vi "statemachine.vi"() -> ()   [LabVIEW 2025]
uses:
  Control 1.ctl
panel:
  out "error in":errorcluster
  out "Enum":T1
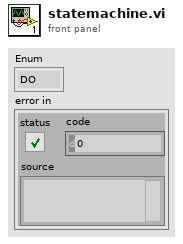
[diagram p1: front panel]
types:
  T1 = typedef "Control 1.ctl" = enum16{"DO", "IDLE", "INIT"}
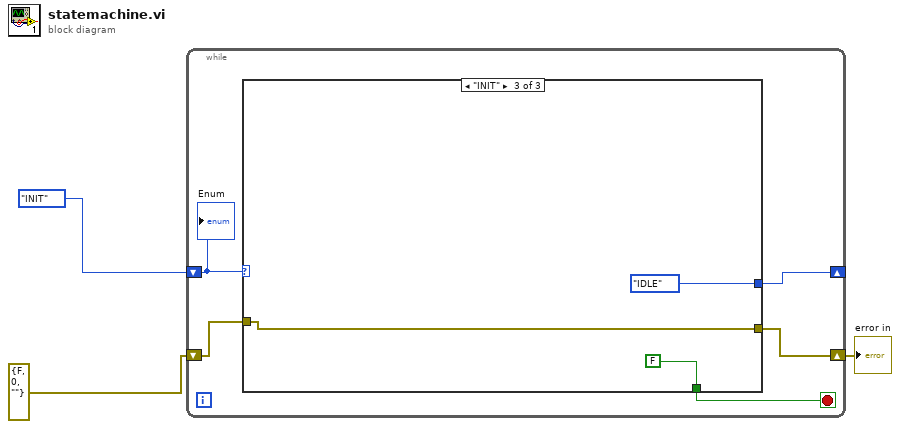
[diagram p0: block diagram]
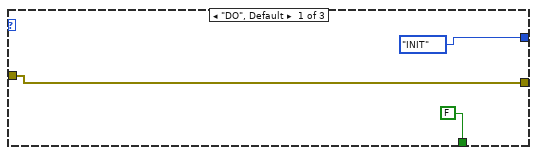
[diagram p2: hidden frame]
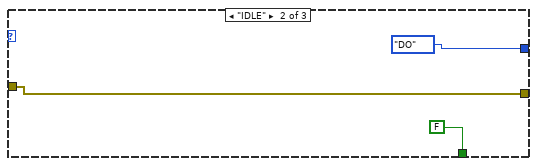
[diagram p3: hidden frame]
diagram:
  n1 = while {
    shift-right: [w8] -> _
    shift-left: Control_1."INIT" ("Enum") -> [w7]
    shift-right: [w5] -> w1
    shift-left: errorcluster {"status"=FALSE, "code"=0, "source"=""} ("error in") -> [w6]
    stop <- w4 stop-if-true
    n2 = case shown="\"INIT\"" w7 {
      tunnel: [Control_1."INIT" ("Enum") Control_1."DO" ("Enum") Control_1."IDLE" ("Enum")] -> w8
      tunnel: w6 -> [w10 w13 w16]
      tunnel: [w10 w13 w16] -> w5
      tunnel: [FALSE FALSE FALSE] -> w4
      frame "DO", Default {
      }
      frame "IDLE" {
      }
      frame "INIT" {
      }
    }
    "Enum" <- w7
  }
  "error in" <- w1
